vi "Debug Screen.vi"() -> ()   [LabVIEW 2013]
uses:
  Common/CL Configuration.ctl
  Common/CL Signal Mapping.ctl
  FPGA/Sector/Accumulate/Sector Parameter Cluster.ctl
  <vilib>/Utility/error.llb/Error Cluster From Error Code.vi
  <vilib>/rvi/errors/niLvFpgaAdjustHostInterfaceError.vi
  <vilib>/rvi/interface/nirviReadWriteControl/nirviReadWriteControl.xnode
  Host/FGs/FPGA_Reference.ctl
  FPGA Bitfiles/8-Tap8-bitCamera_FPGATarget_8-Tap8-bit_Serial_Server.lvbitx
  NiFpgaLv.dll
panel:
  out "Sector Parameters Right":T1
  out "Sector Parameters Left":T1
  out "Analysis Ticks":u32
  out "Acq Control.Initialize":bool
  out "Acq Control.Ignore DVAL 2":bool
  out "Acq Control.Cancel Acq":bool
  out "Acq Control.Acquire 2":bool
  out "Acq Control.Frames To Acq":u32
  out "Acq Control.Line Scan Height":u32
  out "Acq Status.Initialized":bool
  out "Acq Status.DMA Write Timeout":bool
  out "Acq Status.Lines Per Frame":u32
  out "Acq Status.Frames Acq'd":u32
  out "Acq Status.Clocks Per Line":u32
  out "Acq Status.Acq In Progress":bool
  out "# of Frames to Average":u8
  out "CL Config.Signal Mapping":T2
  out "Acq Control.Acquire":bool
  out "CL Config.Configuration":T3
  out "Acq Control.Ignore DVAL":bool
  out "CL Config.Line Scan":bool
  out "CL Config.Spare Active High":bool
  out "CL Config.DVAL Active High":bool
  out "CL Config.LVAL Active High":bool
  out "CL Config.FVAL Active High":bool
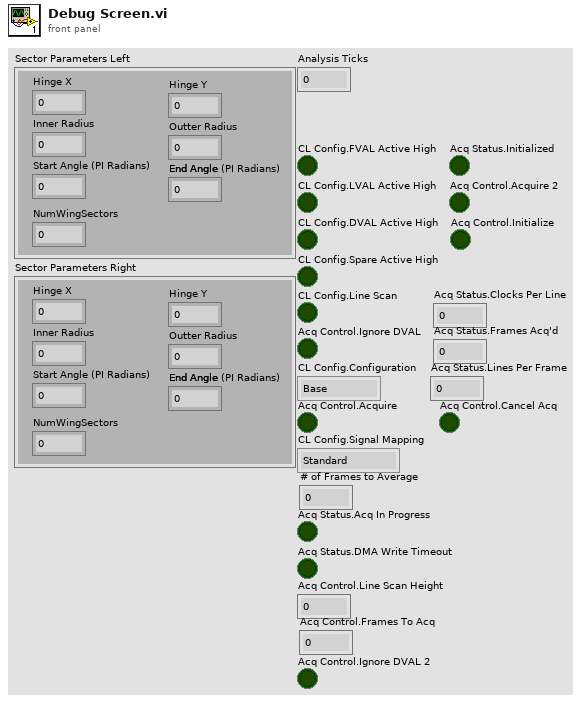
[diagram p1: front panel]
types:
  T1 = typedef "Sector Parameter Cluster.ctl" = cluster{"Start Angle":fxp<+/-,17,2>, "End Angle":fxp<+,17,3>, "Inner Radius":u16, "Outter Radius":u16, "Hinge X":u16, "Hinge Y":u16, "NumWingSectors":u8}
  T2 = typedef "CL Signal Mapping.ctl" = enum8{"Standard", "Basler 10-tap", "Vosskühler 10-tap"}
  T3 = typedef "CL Configuration.ctl" = enum8{"Base", "Medium", "Full"}
  T4 = typedef "FPGA_Reference.ctl" = refnum<k20>
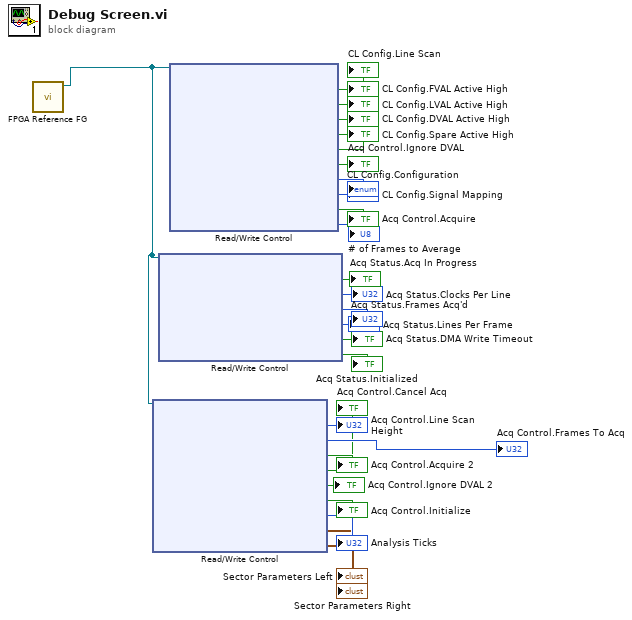
[diagram p0: block diagram]
diagram:
  n1 = call "FPGA Reference FG.vi"() -> ("FPGA VI Reference Out"=w10:T4)  [unwired: 11 in]
  n2 = xnode "Read/Write Control"("FPGA VI Reference In"=w10) -> ("Acq Control.Line Scan Height"=→"Acq Control.Line Scan Height":u32, "Acq Control.Frames To Acq"=→"Acq Control.Frames To Acq":u32, "Acq Control.Acquire"=→"Acq Control.Acquire 2":bool, "Acq Control.Cancel Acq"=→"Acq Control.Cancel Acq":bool, "Acq Control.Ignore DVAL"=→"Acq Control.Ignore DVAL 2":bool, "Acq Control.Initialize"=→"Acq Control.Initialize":bool, "Analysis Ticks"=→"Analysis Ticks":u32, "Sector Parameters Left"=→"Sector Parameters Left":T1, "Sector Parameters Right"=→"Sector Parameters Right":T1)  [unwired: 1 in, 2 out]
  n3 = xnode "Read/Write Control"("FPGA VI Reference In"=w10) -> ("Acq Status.Acq In Progress"=→"Acq Status.Acq In Progress":bool, "Acq Status.Clocks Per Line"=→"Acq Status.Clocks Per Line":u32, "Acq Status.Frames Acq'd"=→"Acq Status.Frames Acq'd":u32, "Acq Status.Lines Per Frame"=→"Acq Status.Lines Per Frame":u32, "Acq Status.DMA Write Timeout"=→"Acq Status.DMA Write Timeout":bool, "Acq Status.Initialized"=→"Acq Status.Initialized":bool)  [unwired: 1 in, 2 out]
  n4 = xnode "Read/Write Control"("FPGA VI Reference In"=w10) -> ("CL Config.FVAL Active High"=→"CL Config.FVAL Active High":bool, "CL Config.LVAL Active High"=→"CL Config.LVAL Active High":bool, "CL Config.DVAL Active High"=→"CL Config.DVAL Active High":bool, "CL Config.Spare Active High"=→"CL Config.Spare Active High":bool, "CL Config.Line Scan"=→"CL Config.Line Scan":bool, "Acq Control.Ignore DVAL"=→"Acq Control.Ignore DVAL":bool, "CL Config.Configuration"=→"CL Config.Configuration":T3, "CL Config.Signal Mapping"=→"CL Config.Signal Mapping":T2, "Acq Control.Acquire"=→"Acq Control.Acquire":bool, "# of Frames to Average"=→"# of Frames to Average":u8)  [unwired: 1 in, 2 out]
